vi "refnums.vi"() -> ()   [LabVIEW 2020]
doc: "This global variable contains refnum names. All refnum names are set in Begin."
panel:
  out "Piston_2":string
  out "Piston_1":string
  out "Piston_0":string
  out "Joystick_Driver":string
  out "Compressor":string
  out "Motor_15":string
  out "Motor_14":string
  out "Motor_13":string
  out "Motor_12":string
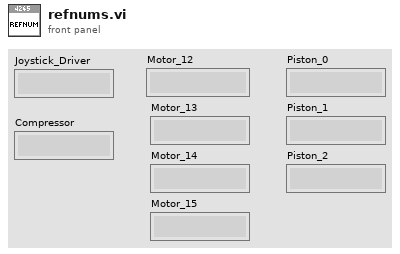
[diagram p1: front panel]
diagram:
